vi "HEWH Rate Averages.vi"(8 "error in (no error)":errorcluster, 9 "Gas Measurment Data":T2, 10 "Gross Heating Value, Vol (Real, Dry)":dbl=1000.0 min=900.0 max=2600.0 step=1.0, 11 "ANSI Rate in":T1) -> (0 "error out":errorcluster, 3 "ANSI Rate out":T1)   [LabVIEW 2020]
uses:
  Range/Type Definitions/RANGE ANSI Rate.ctl
  Drivers/Alicat Gas Meter Driver/Sub-VIs/Data Cluster.ctl
panel:
  # "Totalizer Timer"
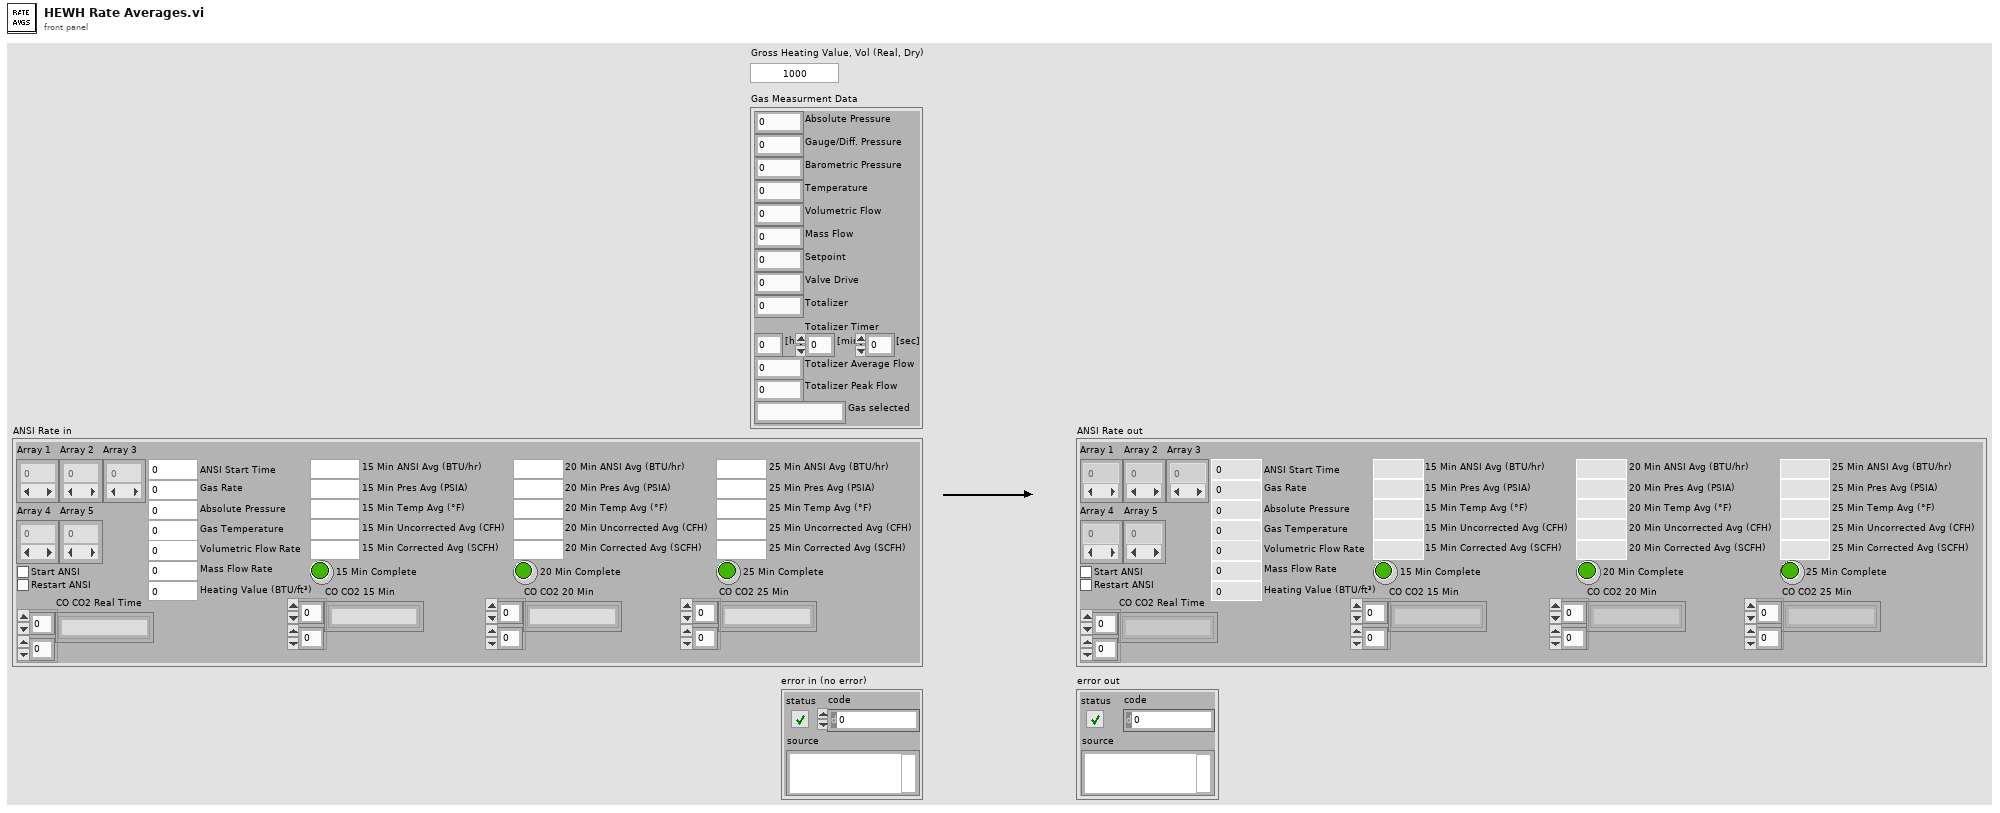
[diagram p1: front panel]
types:
  T1 = typedef "RANGE ANSI Rate.ctl" = cluster{"Array 1":dbl[], "Array 3":dbl[], "Array 2":dbl[], "Start ANSI":bool, "ANSI Start Time":dbl, "Restart ANSI":bool, "15 Min ANSI Avg (BTU/hr)":dbl, "20 Min ANSI Avg (BTU/hr)":dbl, "25 Min ANSI Avg (BTU/hr)":dbl, "Absolute Pressure":dbl, "Gas Temperature":dbl, "Volumetric Flow Rate":dbl, "Mass Flow Rate":dbl, "Array 4":dbl[], "Array 5":dbl[], "Gas Rate":dbl, "15 Min Pres Avg (PSIA)":dbl, "20 Min Pres Avg (PSIA)":dbl, "25 Min Pres Avg (PSIA)":dbl, "15 Min Temp Avg (°F) ":dbl, "20 Min Temp Avg (°F)":dbl, "25 Min Temp Avg (°F)":dbl, "15 Min Uncorrected Avg (CFH)":dbl, "20 Min Uncorrected Avg (CFH)":dbl, "25 Min Uncorrected Avg (CFH)":dbl, "15 Min Corrected Avg (SCFH)":dbl, "20 Min Corrected Avg (SCFH)":dbl, "25 Min Corrected Avg (SCFH)":dbl, "15 Min Complete":bool, "20 Min Complete":bool, "25 Min Complete":bool, "Heating Value (BTU/ft³)":dbl, "CO CO2 15 Min":string[][], "CO CO2 20 Min":string[][], "CO CO2 25 Min":string[][], "CO CO2 Real Time":string[][]}
  T2 = typedef "Data Cluster.ctl" = cluster{"Absolute Pressure":dbl, "Gauge/Diff. Pressure":dbl, "Barometric Pressure":dbl, "Temperature":dbl, "Volumetric Flow":dbl, "Mass Flow":dbl, "Setpoint":dbl, "Valve Drive":dbl, "Totalizer":dbl, "[hr]":dbl, "[min]":dbl, "[sec]":dbl, "Totalizer Average Flow":dbl, "Totalizer Peak Flow":dbl, "Gas selected":string}
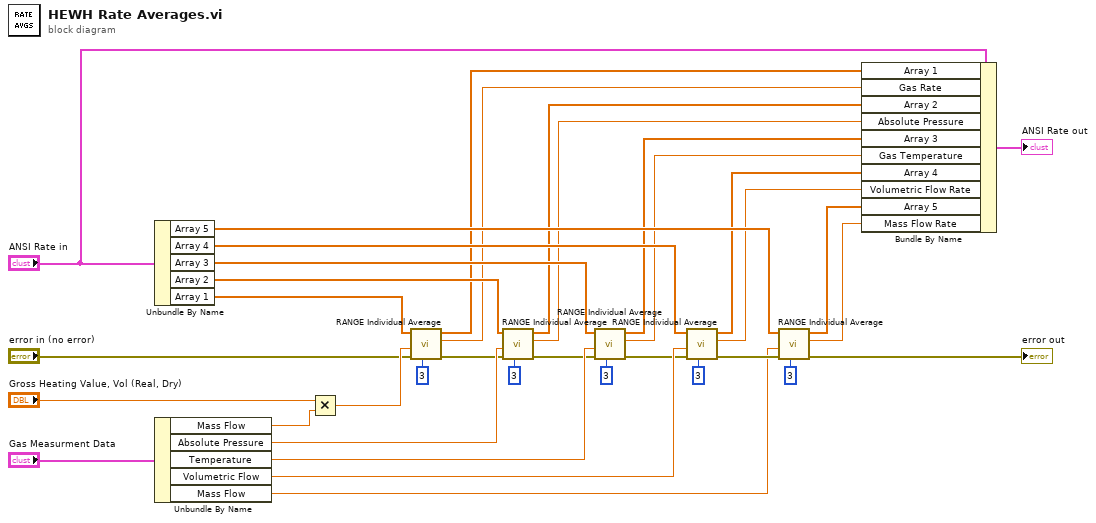
[diagram p0: block diagram]
diagram:
  n1 = Unbundle By Name("ANSI Rate in") -> ("Array 5"=w36:dbl[], "Array 4"=w35:dbl[], "Array 3"=w34:dbl[], "Array 2"=w33:dbl[], "Array 1"=w32:dbl[])
  n2 = Unbundle By Name("Gas Measurment Data") -> ("Mass Flow"=w25:dbl, "Absolute Pressure"=w26:dbl, "Temperature"=w27:dbl, "Volumetric Flow"=w28:dbl, "Mass Flow"=w3:dbl)
  n3 = Multiply(x="Gross Heating Value, Vol (Real, Dry)", y=w25) -> (x*y=w24:dbl)
  n4 = call "RANGE Individual Average.vi"("Avg Interval (Sec)"=3, "Error In"="error in (no error)", "Flow Rate (BTU/HR)"=w24, "Array IN"=w32) -> ("Error Out"=w17:errorcluster, "Average (BTU/HR) (Out)"=w7:dbl, "Array OUT"=w12:dbl[])  [unwired: 4 in, 1 out]
  n5 = call "RANGE Individual Average.vi"("Avg Interval (Sec)"=3, "Error In"=w17, "Flow Rate (BTU/HR)"=w26, "Array IN"=w33) -> ("Error Out"=w18:errorcluster, "Average (BTU/HR) (Out)"=w6:dbl, "Array OUT"=w11:dbl[])  [unwired: 4 in, 1 out]
  n6 = call "RANGE Individual Average.vi"("Avg Interval (Sec)"=3, "Error In"=w18, "Flow Rate (BTU/HR)"=w27, "Array IN"=w34) -> ("Error Out"=w19:errorcluster, "Average (BTU/HR) (Out)"=w5:dbl, "Array OUT"=w10:dbl[])  [unwired: 4 in, 1 out]
  n7 = call "RANGE Individual Average.vi"("Avg Interval (Sec)"=3, "Error In"=w19, "Flow Rate (BTU/HR)"=w28, "Array IN"=w35) -> ("Error Out"=w30:errorcluster, "Average (BTU/HR) (Out)"=w4:dbl, "Array OUT"=w9:dbl[])  [unwired: 4 in, 1 out]
  n8 = call "RANGE Individual Average.vi"("Avg Interval (Sec)"=3, "Error In"=w30, "Flow Rate (BTU/HR)"=w3, "Array IN"=w36) -> ("Error Out"=→"error out":errorcluster, "Average (BTU/HR) (Out)"=w2:dbl, "Array OUT"=w8:dbl[])  [unwired: 4 in, 1 out]
  n9 = Bundle By Name(cluster="ANSI Rate in", "Array 1"=w12, "Gas Rate"=w7, "Array 2"=w11, "Absolute Pressure"=w6, "Array 3"=w10, "Gas Temperature"=w5, "Array 4"=w9, "Volumetric Flow Rate"=w4, "Array 5"=w8, "Mass Flow Rate"=w2) -> (→"ANSI Rate out":T1)
